vi "AnalogDemultiplex_AND.vi"(0 "Analog data cluster":T1) -> (4 "Data A1 out":u64, 6 "Data A2 out":u64)   [LabVIEW 2012]
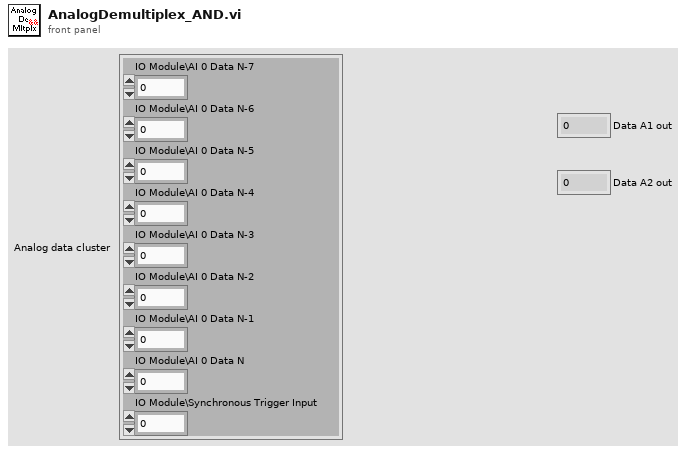
[diagram p1: front panel]
types:
  T1 = cluster{"IO Module\\AI 0 Data N-7":u8, "IO Module\\AI 0 Data N-6":u8, "IO Module\\AI 0 Data N-5":u8, "IO Module\\AI 0 Data N-4":u8, "IO Module\\AI 0 Data N-3":u8, "IO Module\\AI 0 Data N-2":u8, "IO Module\\AI 0 Data N-1":u8, "IO Module\\AI 0 Data N":u8, "IO Module\\Synchronous Trigger Input":u8}
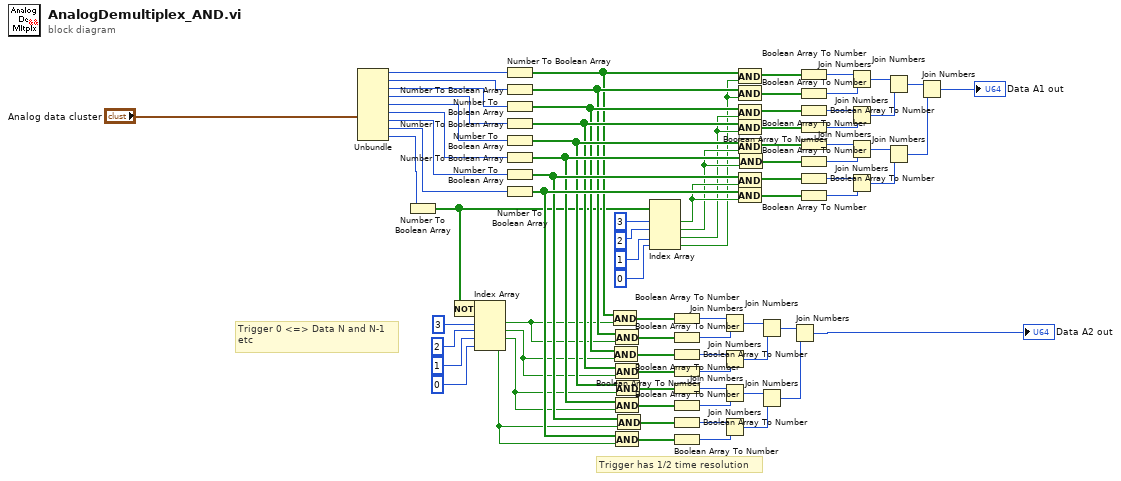
[diagram p0: block diagram]
diagram:
  # "Trigger 0 <=> Data N and N-1\netc"
  # "Trigger has 1/2 time resolution"
  n1 = Unbundle("Analog data cluster") -> ("IO Module\\AI 0 Data N-7"=w22:u8, "IO Module\\AI 0 Data N-6"=w21:u8, "IO Module\\AI 0 Data N-5"=w20:u8, "IO Module\\AI 0 Data N-4"=w19:u8, "IO Module\\AI 0 Data N-3"=w18:u8, "IO Module\\AI 0 Data N-2"=w17:u8, "IO Module\\AI 0 Data N-1"=w16:u8, "IO Module\\AI 0 Data N"=w15:u8, "IO Module\\Synchronous Trigger Input"=w14:u8)
  n2 = Number To Boolean Array(number=w14) -> (Boolean array=w45:bool[])
  n3 = Not(x=w45) -> (.not. x?=w46:bool[])
  n4 = Index Array(array=w46, index #1=3 ("index"), index #2=2 ("index"), index #3=1 ("index"), index #4=0 ("index")) -> (element #1=w61:bool, element #2=w62:bool, element #3=w63:bool, element #4=w64:bool)
  n5 = Number To Boolean Array(number=w22) -> (Boolean array=w65:bool[])
  n6 = Number To Boolean Array(number=w21) -> (Boolean array=w66:bool[])
  n7 = Number To Boolean Array(number=w20) -> (Boolean array=w67:bool[])
  n8 = Number To Boolean Array(number=w19) -> (Boolean array=w68:bool[])
  n9 = Number To Boolean Array(number=w18) -> (Boolean array=w69:bool[])
  n10 = Number To Boolean Array(number=w17) -> (Boolean array=w70:bool[])
  n11 = Number To Boolean Array(number=w16) -> (Boolean array=w71:bool[])
  n12 = Number To Boolean Array(number=w15) -> (Boolean array=w72:bool[])
  n13 = And(x=w65, y=w61) -> (x .and. y?=w73:bool[])
  n14 = And(x=w67, y=w62) -> (x .and. y?=w75:bool[])
  n15 = And(x=w66, y=w61) -> (x .and. y?=w74:bool[])
  n16 = And(x=w68, y=w62) -> (x .and. y?=w76:bool[])
  n17 = And(x=w70, y=w63) -> (x .and. y?=w78:bool[])
  n18 = And(x=w72, y=w64) -> (x .and. y?=w80:bool[])
  n19 = And(x=w69, y=w63) -> (x .and. y?=w77:bool[])
  n20 = And(x=w71, y=w64) -> (x .and. y?=w79:bool[])
  n21 = Index Array(array=w45, index #1=3 ("index"), index #2=2 ("index"), index #3=1 ("index"), index #4=0 ("index")) -> (element #1=w4:bool, element #2=w3:bool, element #3=w2:bool, element #4=w1:bool)
  n22 = Boolean Array To Number(Boolean array=w73) -> (number=w53:u8)
  n23 = Boolean Array To Number(Boolean array=w74) -> (number=w54:u8)
  n24 = Boolean Array To Number(Boolean array=w75) -> (number=w55:u8)
  n25 = Boolean Array To Number(Boolean array=w76) -> (number=w56:u8)
  n26 = Boolean Array To Number(Boolean array=w77) -> (number=w57:u8)
  n27 = Boolean Array To Number(Boolean array=w78) -> (number=w58:u8)
  n28 = Boolean Array To Number(Boolean array=w79) -> (number=w59:u8)
  n29 = Boolean Array To Number(Boolean array=w80) -> (number=w60:u8)
  n30 = Join Numbers(hi=w53, lo=w54) -> ((hi.lo)=w47:u16)
  n31 = Join Numbers(hi=w55, lo=w56) -> ((hi.lo)=w48:u16)
  n32 = Join Numbers(hi=w57, lo=w58) -> ((hi.lo)=w49:u16)
  n33 = Join Numbers(hi=w59, lo=w60) -> ((hi.lo)=w50:u16)
  n34 = And(x=w65, y=w1) -> (x .and. y?=w29:bool[])
  n35 = And(x=w66, y=w1) -> (x .and. y?=w31:bool[])
  n36 = And(x=w67, y=w2) -> (x .and. y?=w32:bool[])
  n37 = And(x=w68, y=w2) -> (x .and. y?=w33:bool[])
  n38 = And(x=w69, y=w3) -> (x .and. y?=w34:bool[])
  n39 = And(x=w71, y=w4) -> (x .and. y?=w36:bool[])
  n40 = And(x=w72, y=w4) -> (x .and. y?=w37:bool[])
  n41 = And(x=w70, y=w3) -> (x .and. y?=w35:bool[])
  n42 = Join Numbers(hi=w47, lo=w48) -> ((hi.lo)=w52:u32)
  n43 = Join Numbers(hi=w49, lo=w50) -> ((hi.lo)=w51:u32)
  n44 = Join Numbers(hi=w52, lo=w51) -> ((hi.lo)=→"Data A2 out":u64)
  n45 = Boolean Array To Number(Boolean array=w29) -> (number=w30:u8)
  n46 = Boolean Array To Number(Boolean array=w31) -> (number=w38:u8)
  n47 = Boolean Array To Number(Boolean array=w32) -> (number=w39:u8)
  n48 = Boolean Array To Number(Boolean array=w33) -> (number=w40:u8)
  n49 = Boolean Array To Number(Boolean array=w34) -> (number=w41:u8)
  n50 = Boolean Array To Number(Boolean array=w35) -> (number=w42:u8)
  n51 = Boolean Array To Number(Boolean array=w36) -> (number=w43:u8)
  n52 = Boolean Array To Number(Boolean array=w37) -> (number=w44:u8)
  n53 = Join Numbers(hi=w30, lo=w38) -> ((hi.lo)=w23:u16)
  n54 = Join Numbers(hi=w39, lo=w40) -> ((hi.lo)=w24:u16)
  n55 = Join Numbers(hi=w41, lo=w42) -> ((hi.lo)=w25:u16)
  n56 = Join Numbers(hi=w43, lo=w44) -> ((hi.lo)=w26:u16)
  n57 = Join Numbers(hi=w23, lo=w24) -> ((hi.lo)=w28:u32)
  n58 = Join Numbers(hi=w25, lo=w26) -> ((hi.lo)=w27:u32)
  n59 = Join Numbers(hi=w28, lo=w27) -> ((hi.lo)=→"Data A1 out":u64)
